vi "Stop_current_SciScan.vi"(8 "error in (no error)":errorcluster, 11 "Current SciScan":string) -> (0 "error out":errorcluster)   [LabVIEW 2012]
uses:
  GFG/GFG Translator Wrapper/GFGTranslator_Action.ctl
  GFG/GFG Translator Wrapper/GFGTranslator_Datatype.ctl
  GFG/GFG Translator Wrapper/GFGTranslator_errors.ctl
  <vilib>/DAQmx/create/channels.llb/DAQmx Create Channel (AO-Voltage-Basic).vi
  <vilib>/DAQmx/write.llb/DAQmx Write (Analog DBL 1Chan 1Samp).vi
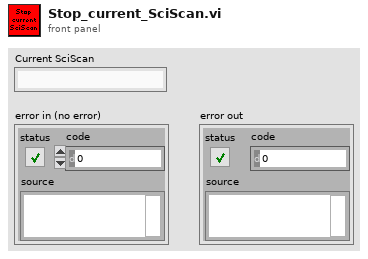
[diagram p1: front panel]
types:
  T1 = typedef "GFGTranslator_Datatype.ctl" = enum16{"String", "Path (String)", "Numeric", "Boolean", "Set_BoolRef (use boolean data)", "Get_Variant", "Get_2DArray (I16)", "Get_Image_2DArray (I16)", "Get_Version (String)", "Get_All GFG variables (String)"}
  T2 = typedef "GFGTranslator_Action.ctl" = enum16{"Get", "Set"}
  T3 = typedef "GFGTranslator_errors.ctl" = enum16{"Success", "SciScan Not Running", "No Get Method for Selected Datatype", "No Set Method for Selected Datatype", "Variable Not Found", "Unexpected Datatype", "Data Out of Range"}
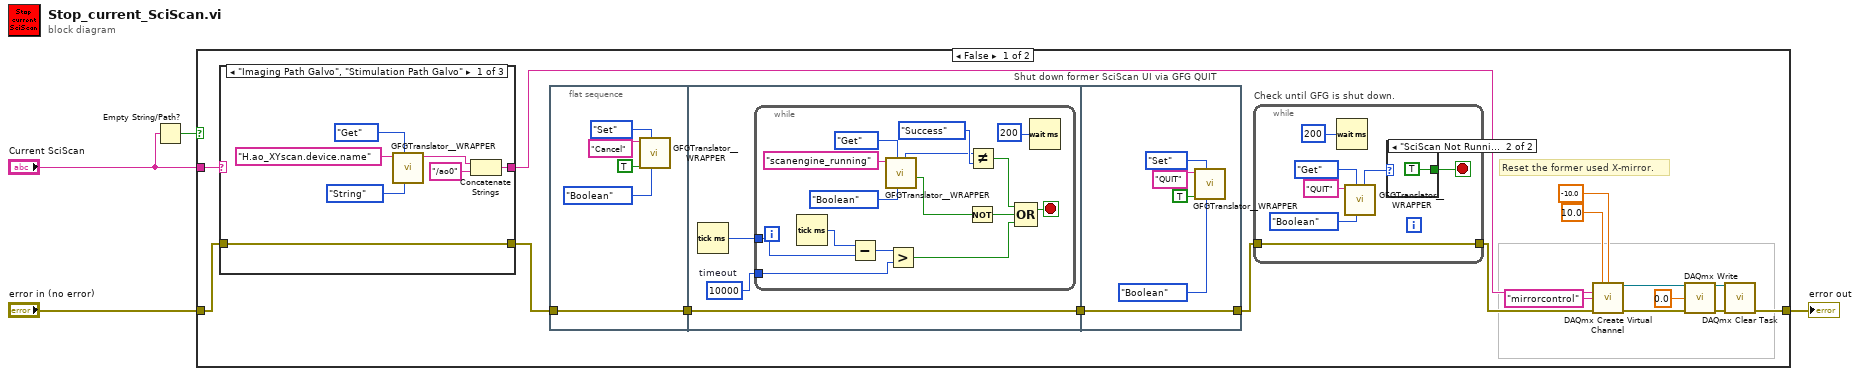
[diagram p0: block diagram]
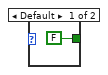
[diagram p2: hidden frame]
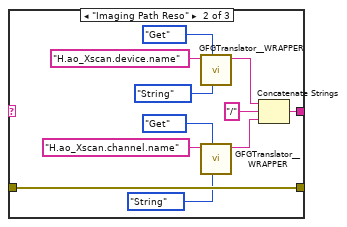
[diagram p3: hidden frame]
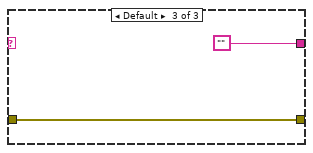
[diagram p4: hidden frame]
diagram:
  n1 = Empty String/Path?(string/path="Current SciScan") -> (empty?=w1:bool)
  n2 = case shown="False" w1 {
    tunnel: "Current SciScan" -> [w21 _]
    tunnel: "error in (no error)" -> [w20 w79]
    tunnel: [w19 w79] -> w3
    frame False {
      # "Reset the former used X-mirror."
      n3 = case shown="\"Imaging Path Galvo\", \"Stimulation Path Galvo\"" w21 {
        tunnel: [w59 w66 ""] -> w17
        tunnel: w20 -> [w62 w73 w77]
        tunnel: [w62 w73 w77] -> w18
        frame "Imaging Path Galvo", "Stimulation Path Galvo" {
          n4 = call "GFGTranslator__WRAPPER.vi"("GFGTranslator Datatype"=GFGTranslator_Datatype."String", "GFG Translator Action"=GFGTranslator_Action."Get", "GFG Variable Name"="H.ao_XYscan.device.name" ("Variable Name in")) -> ("String_Output"=w61:string)  [unwired: 3 in, 5 out]
          n5 = Concatenate Strings(w61, "/ao0" ("string")) -> (w59:string)
        }
        frame "Imaging Path Reso" {
          n6 = call "GFGTranslator__WRAPPER.vi"("GFGTranslator Datatype"=GFGTranslator_Datatype."String", "GFG Translator Action"=GFGTranslator_Action."Get", "GFG Variable Name"="H.ao_Xscan.device.name" ("Variable Name in")) -> ("String_Output"=w69:string)  [unwired: 3 in, 5 out]
          n7 = call "GFGTranslator__WRAPPER.vi"("GFGTranslator Datatype"=GFGTranslator_Datatype."String", "GFG Translator Action"=GFGTranslator_Action."Get", "GFG Variable Name"="H.ao_Xscan.channel.name" ("Variable Name in")) -> ("String_Output"=w67:string)  [unwired: 3 in, 5 out]
          n8 = Concatenate Strings(w69, "/" ("String_Output"), w67) -> (w66:string)
        }
        frame Default {
        }
      }
      n9 = flat-sequence "Shut down former SciScan UI via GFG QUIT" {
        tunnel: w18 -> [w26]
        tunnel: [w26] -> w5
        tunnel: [w29] -> w6
        tunnel: w5 -> [w29]
        tunnel: [w45] -> w8
        tunnel: w6 -> [w45]
        frame #0 {
          n10 = call "GFGTranslator__WRAPPER.vi"("GFGTranslator Datatype"=GFGTranslator_Datatype."Boolean", "GFG Translator Action"=GFGTranslator_Action."Set", "Boolean_Input"=TRUE, "GFG Variable Name"="Cancel") -> ()  [unwired: 2 in, 6 out]
        }
        frame #1 {
          w27 = u32 10000  # timeout
          n11 = Tick Count (ms)() -> (millisecond timer value=w28:u32)
          n12 = while {
            tunnel: w28 -> [w33]
            tunnel: w27 -> [w31]
            stop <- w39 stop-if-true
            n13 = Tick Count (ms)() -> (millisecond timer value=w34:u32)
            n14 = Subtract(x=w34, y=w33) -> (x-y=w32:u32)
            n15 = call "GFGTranslator__WRAPPER.vi"("GFGTranslator Datatype"=GFGTranslator_Datatype."Boolean", "GFG Translator Action"=GFGTranslator_Action."Get", "GFG Variable Name"="scanengine_running") -> ("Boolean_Output"=w40:bool, "Status Output"=w37:T3)  [unwired: 3 in, 4 out]
            n16 = Greater?(x=w32, y=w31) -> (0:w30:bool)
            n17 = Not(x=w40) -> (.not. x?=w35:bool)
            n18 = Not Equal?(x=w37, y=GFGTranslator_errors."Success" ("Status Output")) -> (x != y?=w36:bool)
            n19 = Compound Arithmetic op=OR(w36, w35, w30) -> (w39:bool)
            n20 = Wait (ms)(milliseconds to wait=u32 200) -> ()  [unwired: 1 out]
          }
        }
        frame #2 {
          n21 = call "GFGTranslator__WRAPPER.vi"("GFGTranslator Datatype"=GFGTranslator_Datatype."Boolean", "GFG Translator Action"=GFGTranslator_Action."Set", "Boolean_Input"=TRUE, "GFG Variable Name"="QUIT") -> ()  [unwired: 2 in, 6 out]
        }
      }
      n22 = while "Check until GFG is shut down." {
        tunnel: w8 -> [w51]
        tunnel: [w51] -> w14
        stop <- w54 stop-if-true
        n23 = Wait (ms)(milliseconds to wait=u32 200) -> ()  [unwired: 1 out]
        n24 = call "GFGTranslator__WRAPPER.vi"("GFGTranslator Datatype"=GFGTranslator_Datatype."Boolean", "GFG Translator Action"=GFGTranslator_Action."Get", "GFG Variable Name"="QUIT") -> ("Status Output"=w55:T3)  [unwired: 3 in, 5 out]
        n25 = case shown="\"SciScan Not Running\"" w55 {
          tunnel: [FALSE TRUE] -> w54
          frame Default {
          }
          frame "SciScan Not Running" {
          }
        }
      }
      n26 = call-poly <vilib>:"DAQmx Create Virtual Channel.vi"("maximum value"=10.0, "minimum value"=-10.0 ("maximum value"), "physical channels"=w17, "name to assign"="mirrorcontrol", "error in"=w14) -> ("task out"=w11:refnum<k21>, "error out"=w15:errorcluster)  [unwired: 9 in]
      n27 = call-poly <vilib>:"DAQmx Write.vi"("task/channels in"=w11, "data"=0.0, "error in"=w15) -> ("task out"=w13:refnum<k21>, "error out"=w16:errorcluster)  [unwired: 10 in, 1 out]
      n28 = call <vilib>:"DAQmx Clear Task.vi"("task in"=w13, "error in"=w16) -> ("error out"=w19:errorcluster)  [unwired: 13 in]
    }
    frame True {
    }
  }
  "error out" <- w3
